vi "读取固件状态.vi"(8 "错误输入":errorcluster, 11 "MB session in":refnum<class "MB_Master.lvclass">) -> (0 "error out":errorcluster, 1 "固件状态":enum16{"正常", "砖头"}(ring), 2 "结果字符串":string, 3 "MB session out":refnum<class "MB_Master.lvclass">)   [LabVIEW 2016, in "斯坦道总氮.lvlib"]
uses:
  <vilib>/Plasmionique/MB Master/MB_Master/MB_Master.lvclass
  <vilib>/Plasmionique/MB Master/MB_Master_Serial/MB_Master_Serial.lvclass
  C:/Program Files (x86)/National Instruments/LabVIEW 2016/vi.lib/Plasmionique/MB Master/MB_Master/MB_Master.lvclass
  <vilib>/Plasmionique/MB Master/MB Master.lvlib
panel:
  in  "VISA Resource":refnum<visa-resource-name>
  in  "引用选择":enum16{"MB引用", "自建引用"}(ring)
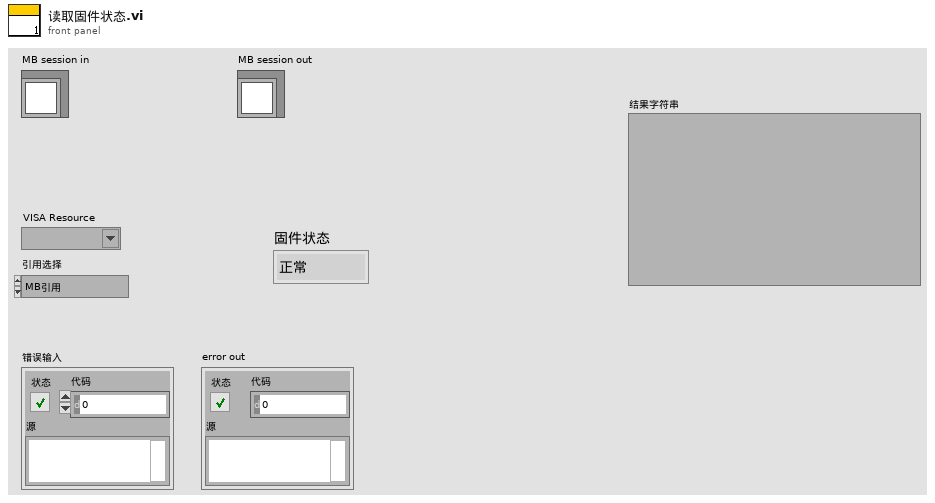
[diagram p1: front panel]
types:
  T1 = cluster{"baud rate (bps)":u32, "stop bits":u16, "parity":u16, "flow control":u16, "timeout":u32, "retries":i32}
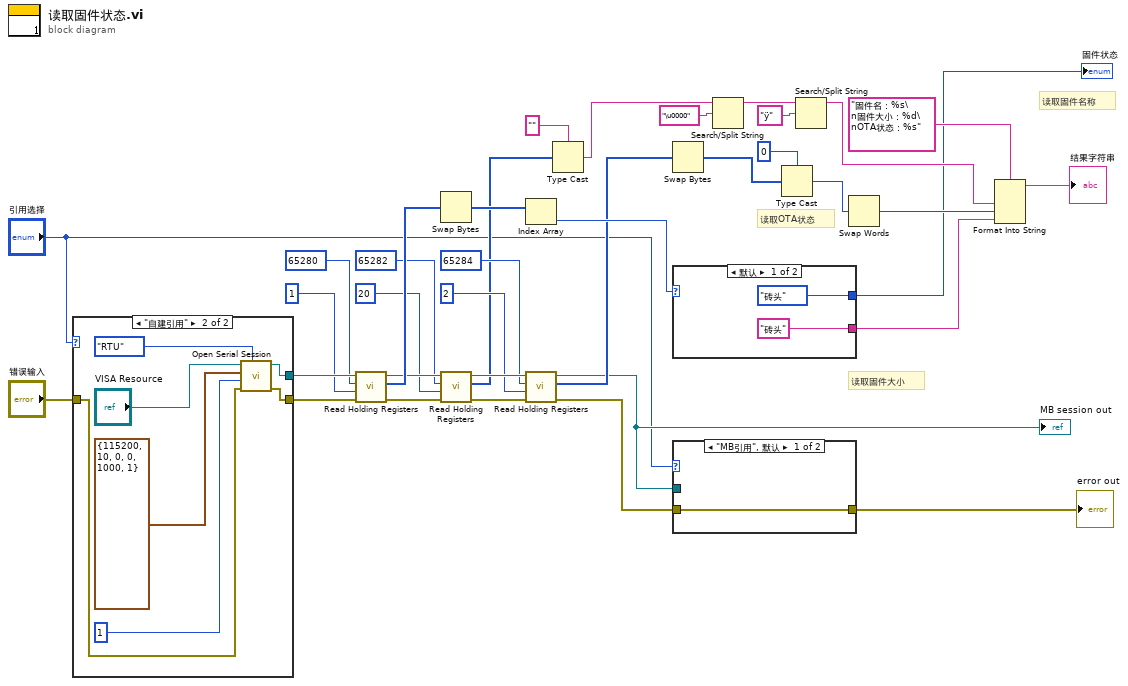
[diagram p0: block diagram]
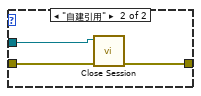
[diagram p2: hidden frame]
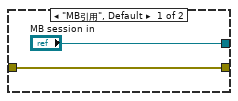
[diagram p3: hidden frame]
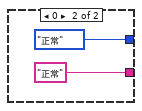
[diagram p4: hidden frame]
diagram:
  # "读取固件大小"
  # "读取固件名称"
  # "读取OTA状态"
  n1 = case shown="\"自建引用\"" "引用选择" {
    tunnel: ["MB session in" w44] -> w35
    tunnel: "错误输入" -> [w37 w43]
    tunnel: [w37 w42] -> w14
    frame "MB引用", Default {
    }
    frame "自建引用" {
      n2 = call <vilib>:"Open Serial Session.vi"("Mode (RTU)"=enum16{"RTU", "ASCII"}."RTU", "Error in"=w43, "Slave ID"=u8 1, "Serial Config"=T1 {"baud rate (bps)"=115200, "stop bits"=10, "parity"=0, "flow control"=0, "timeout"=1000, "retries"=1}, "VISA Resource"="VISA Resource") -> ("Error out"=w42:errorcluster, "MB_Serial session"=w44:refnum<class "MB_Master_Serial.lvclass">)  [unwired: 5 in]
    }
  }
  n3 = call <vilib>:"Read Holding Registers.vi"("error in (no error)"=w14, "quantity"=u16 1, "starting address"=u16 65280, "MB session in"=w35) -> ("error out"=w22:errorcluster, "Registers"=w32:u16[], "MB session out"=w27:refnum<class "MB_Master.lvclass">)  [unwired: 5 in]
  n4 = Swap Bytes(anything=w32) -> (byte swapped=w30:u16[])
  n5 = call <vilib>:"Read Holding Registers.vi"("error in (no error)"=w22, "quantity"=u16 20, "starting address"=u16 65282, "MB session in"=w27) -> ("error out"=w21:errorcluster, "Registers"=w9:u16[], "MB session out"=w25:refnum<class "MB_Master.lvclass">)  [unwired: 5 in]
  n6 = Index Array(array=w30) -> (element=w31:u16)  [unwired: 1 in]
  n7 = call <vilib>:"Read Holding Registers.vi"("error in (no error)"=w21, "quantity"=u16 2, "starting address"=u16 65284, "MB session in"=w25) -> ("error out"=w7:errorcluster, "Registers"=w20:u16[], "MB session out"=w8:refnum<class "MB_Master.lvclass">)  [unwired: 5 in]
  "MB session out" <- w8
  n8 = Type Cast(type="", x=w9) -> (*(type *) &x=w10:string)
  n9 = Swap Bytes(anything=w20) -> (byte swapped=w19:u16[])
  n10 = case shown="默认" w31 {
    tunnel: ["砖头" "正常"] -> w29
    tunnel: [enum16{"正常", "砖头"}."砖头" ("固件状态") enum16{"正常", "砖头"}."正常" ("固件状态")] -> w1
    frame Default {
    }
    frame 0 {
    }
  }
  "固件状态" <- w1
  n11 = case shown="\"MB引用\", 默认" "引用选择" {
    tunnel: w8 -> [_ w53]
    tunnel: w7 -> [w50 w52]
    tunnel: [w50 w51] -> w6
    frame "MB引用", Default {
    }
    frame "自建引用" {
      n12 = call-dynamic "Close Session.vi"("error in (no error)"=w52, "MB session in"=w53) -> ("error out"=w51:errorcluster)  [unwired: 9 in]
    }
  }
  "error out" <- w6
  n13 = Search/Split String(string=w10, search string/char (-)="\u0000" ("搜索字符串")) -> (substring before match=w4:string)  [unwired: 1 in, 2 out]
  n14 = Type Cast(type=u32 0, x=w19) -> (*(type *) &x=w17:u32)
  n15 = Search/Split String(string=w4, search string/char (-)="ÿ" ("搜索字符串")) -> (substring before match=w3:string)  [unwired: 1 in, 2 out]
  n16 = Swap Words(1:w17) -> (0:w16:u32)
  n17 = Format Into String(format string="固件名：%s\n固件大小：%d\nOTA状态：%s" ("格式字符串"), w3, w16, w29) -> (resulting string=→"结果字符串":string)  [unwired: 2 in, 1 out]
